vi "FilterSet.vi"(8 "error in (no error)":errorcluster caption="错误输入（无错误）", 11 "ParamIn":cluster{"mode":u8, "AccCode":u32, "AccMask":u32}={"mode"=1, "AccCode"=0, "AccMask"=4294967295} {"AccMask" format="%08x"; "AccCode" format="%08x"; "mode" items=["接收所有类型"=1, "只接收标准帧"=2, "只接收扩展帧"=3]}) -> (0 "error out":errorcluster caption="错误输出", 2 "Cancel？":bool, 3 "ParamOut":cluster{"mode":u8, "AccCode":u32, "AccMask":u32}={"mode"=1, "AccCode"=0, "AccMask"=0} {"AccMask" format="%08x"; "AccCode" format="%08x"; "mode" items=["接收所有类型"=1, "只接收标准帧"=2, "只接收扩展帧"=3]})   [LabVIEW 2011]
doc: "ID=0x6006"
panel:
  out "label2":string="CAN中继状态"
  in  "calc":bool
  in  "cancel":bool
  in  "ok":bool
  in  "AccMask":u32 caption="ÆÁ±Î´a£º0x" format="%08x"
  in  "AccCode":u32 caption="òžÊÕ´a£º0x" format="%08x"
  in  "mode":u8(ring)=1 caption="濾波方式:" items=["接收所有類型"=1, "Ö»ÊÕ˜ËœÊŽ¬"=2, "Ö»ÊÕ”UÕ¹Ž¬"=3]
  in  "selfdef":bool
  out "tab":enum32{"标准ID", "扩展ID", "全ID"}(tab)
  in  "ID00":bool
  in  "ID01":bool
  in  "ID02":bool
  in  "ID03":bool
  in  "ID04":bool
  in  "ID05":bool
  in  "ID06":bool
  in  "ID07":bool
  in  "ID08":bool
  in  "ID09":bool
  in  "ID10":bool
  in  "t1":i32(listbox)=-1
  in  "EID17":bool
  in  "EID16":bool
  in  "EID15":bool
  in  "EID14":bool
  in  "EID13":bool
  in  "EID12":bool
  in  "EID11":bool
  in  "EID10":bool
  in  "EID09":bool
  in  "EID08":bool
  in  "EID07":bool
  in  "EID06":bool
  in  "EID05":bool
  in  "EID04":bool
  in  "EID03":bool
  in  "EID02":bool
  in  "EID01":bool
  in  "EID00":bool
  in  "EID26":bool
  in  "EID25":bool
  in  "EID24":bool
  in  "EID23":bool
  in  "EID22":bool
  in  "EID21":bool
  in  "EID20":bool
  in  "EID19":bool
  in  "EID18":bool
  in  "EID27":bool
  in  "EID28":bool
  in  "t2":i32(listbox)=-1
  in  "ID10 2":bool
  in  "ID09 2":bool
  in  "ID08 2":bool
  in  "ID07 2":bool
  in  "ID06 2":bool
  in  "ID05 2":bool
  in  "ID04 2":bool
  in  "ID03 2":bool
  in  "ID02 2":bool
  in  "ID01 2":bool
  in  "ID00 2":bool
  in  "EID17 2":bool
  in  "EID16 2":bool
  in  "EID15 2":bool
  in  "EID14 2":bool
  in  "EID13 2":bool
  in  "EID12 2":bool
  in  "EID11 2":bool
  in  "EID10 2":bool
  in  "EID09 2":bool
  in  "EID08 2":bool
  in  "EID07 2":bool
  in  "EID06 2":bool
  in  "EID05 2":bool
  in  "EID04 2":bool
  in  "EID03 2":bool
  in  "EID02 2":bool
  in  "EID01 2":bool
  in  "EID00 2":bool
  in  "EID26 2":bool
  in  "EID25 2":bool
  in  "EID24 2":bool
  in  "EID23 2":bool
  in  "EID22 2":bool
  in  "EID21 2":bool
  in  "EID20 2":bool
  in  "EID19 2":bool
  in  "EID18 2":bool
  in  "EID27 2":bool
  in  "EID28 2":bool
  in  "t3":i32(listbox)=-1
  in  "Submit":bool
  in  "IDSet":u32 caption="指定ID：0x" format="%x"
  in  "FilterMode":u16(ring) caption="žV²¨Ä£Ê½ßx“ñ£º" items=["½ÓÊÕËùÓÐ”µ“þ", "˜ËœÊŽ¬žV²¨£¨ÔO¶¨½ÓÊÕ†Î‚€ID£©", "”UÕ¹Ž¬žV²¨£¨ÔO¶¨½ÓÊÕ†Î‚€ID£©", "˜ËœÊŽ¬žV²¨£¨ƒHID£¬×ÔÓÉÔO¶¨£©", "”UÕ¹Ž¬žV²¨£¨ƒHID£¬×ÔÓÉÔO¶¨£©"]
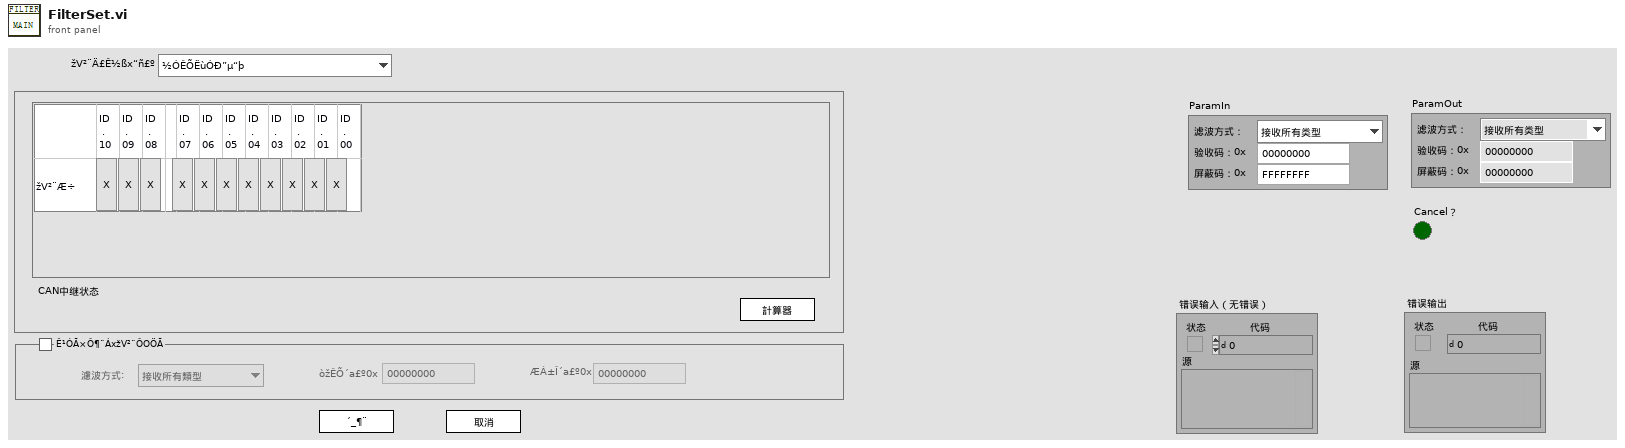
[diagram p1: front panel]
types:
  T1 = cluster{"FilterMode":refnum<vi>, "IDSet":refnum<vi>, "t1":refnum<vi>, "t2":refnum<vi>, "t3":refnum<vi>, "Submit":refnum<vi>, "tab":refnum<vi>, "calc":refnum<vi>, "selfdef":refnum<vi>, "mode":refnum<vi>, "AccCode":refnum<vi>, "AccMask":refnum<vi>, "ok":refnum<vi>, "cancel":refnum<vi>}
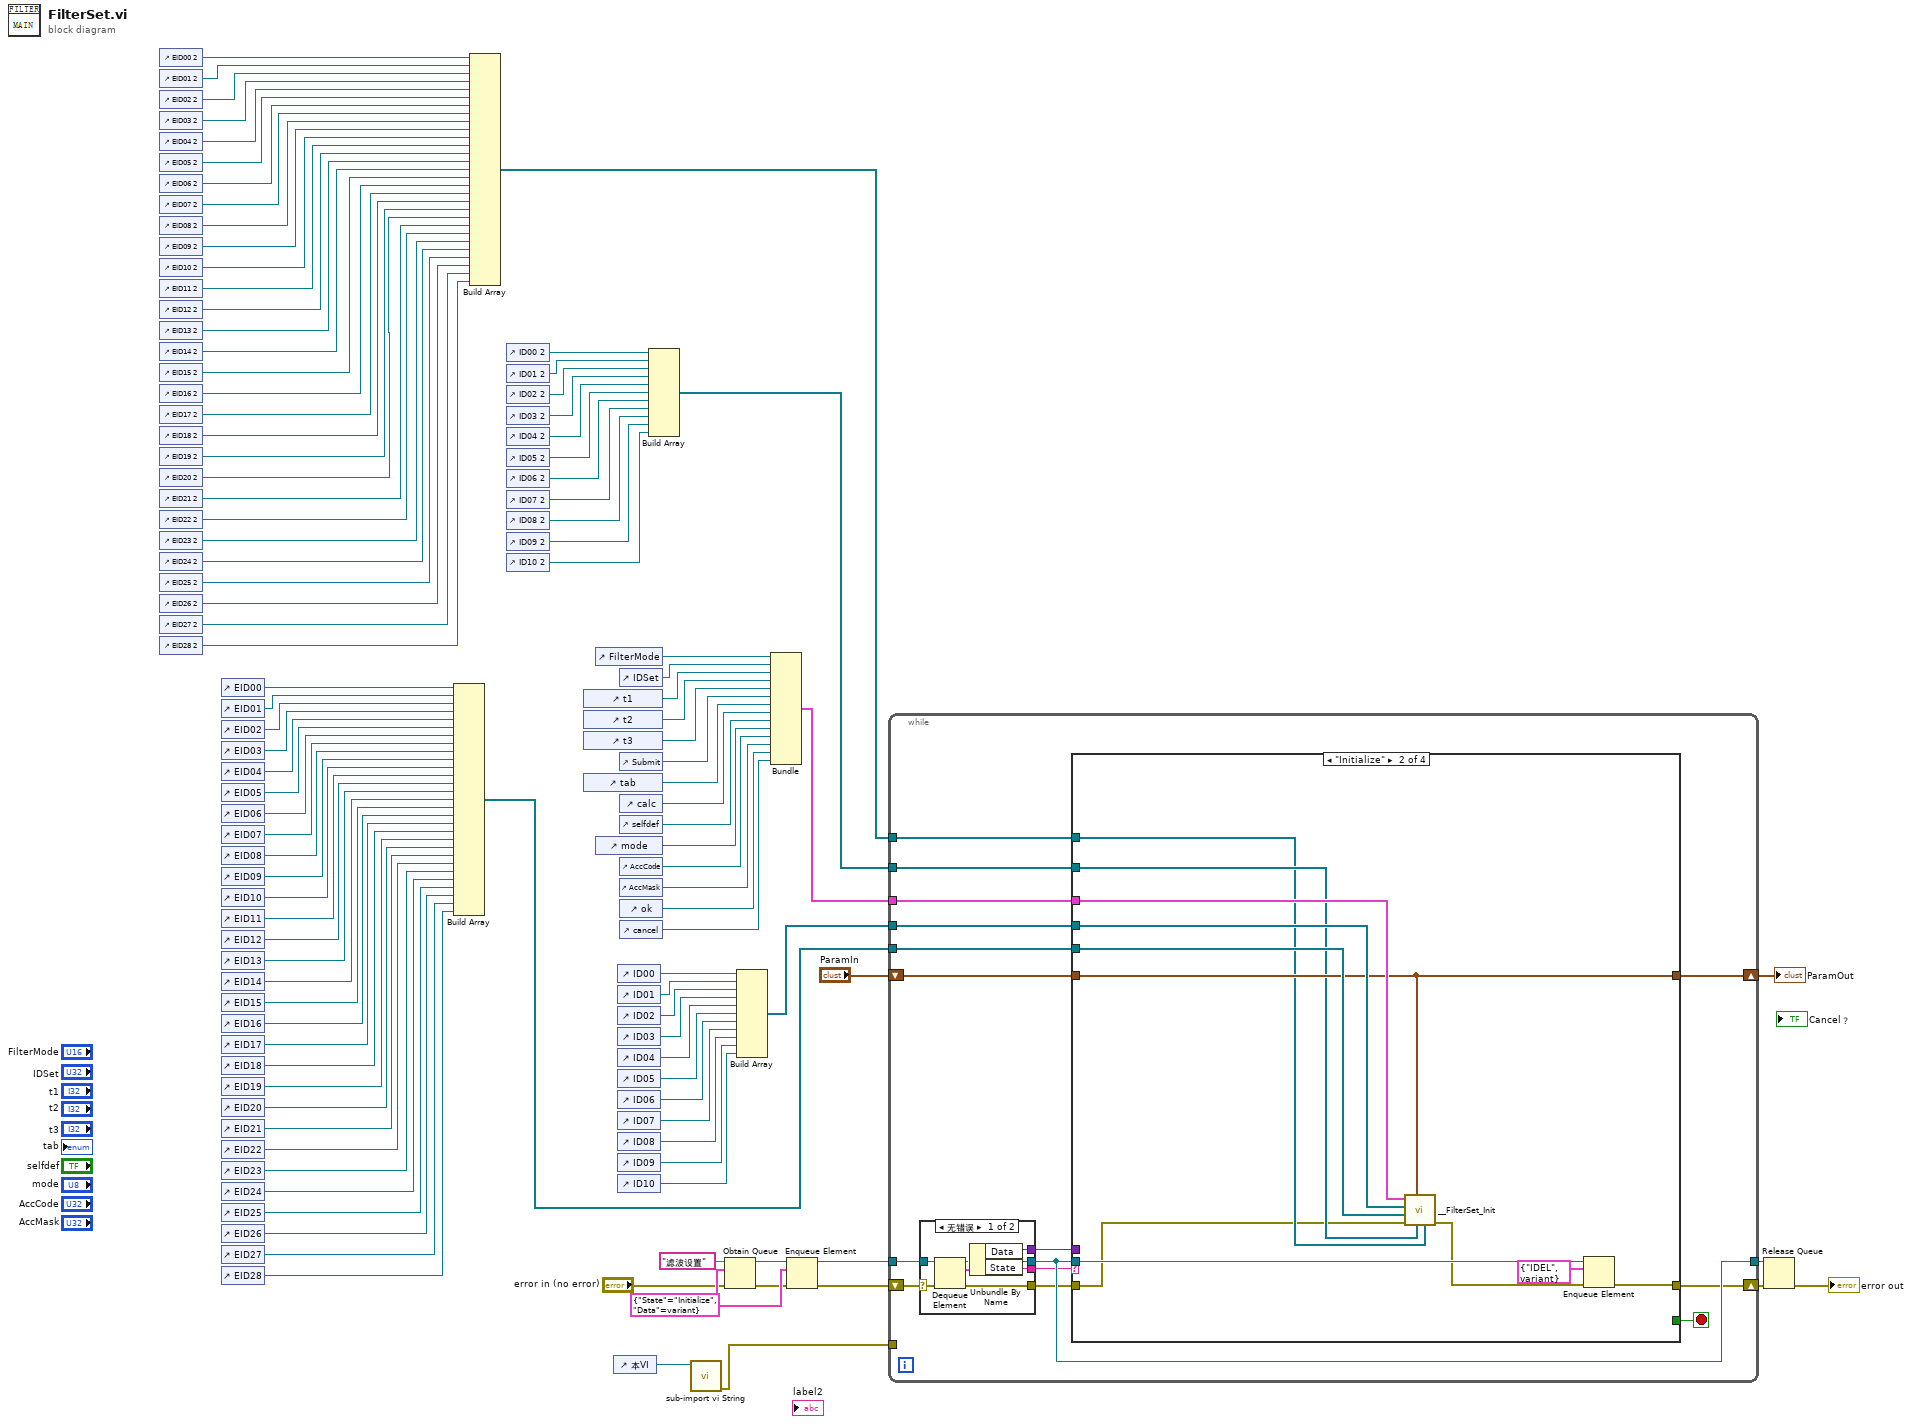
[diagram p0: block diagram]
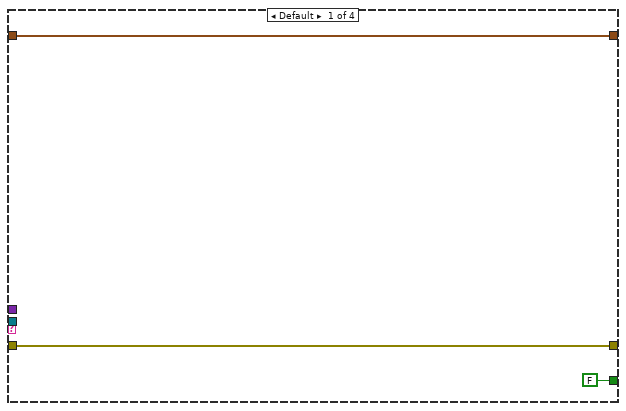
[diagram p2: hidden frame]
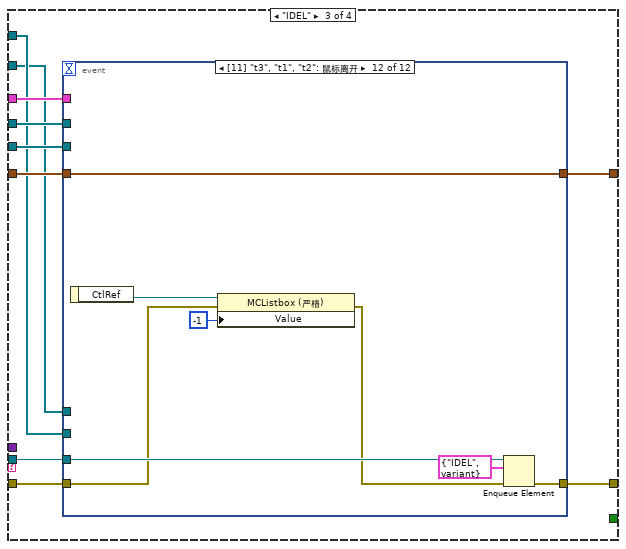
[diagram p3: hidden frame]
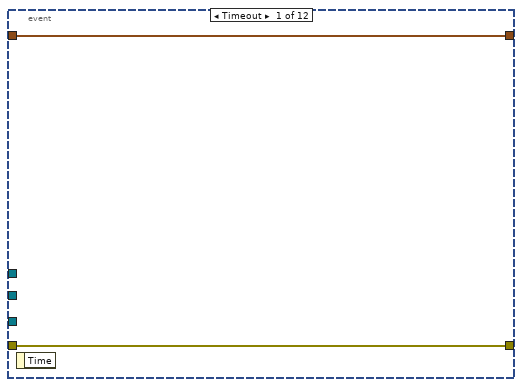
[diagram p4: hidden frame]
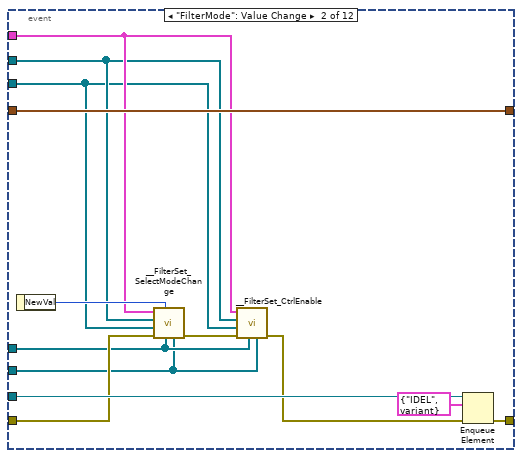
[diagram p5: hidden frame]
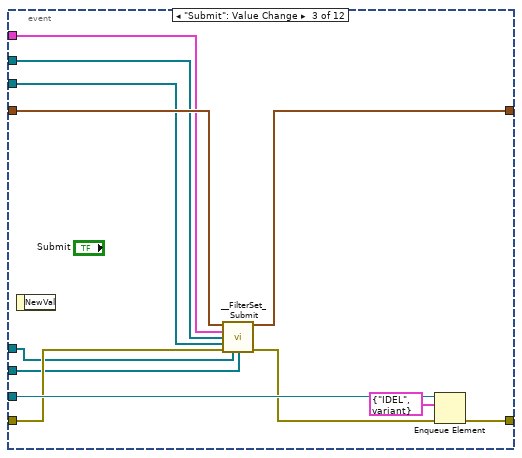
[diagram p6: hidden frame]
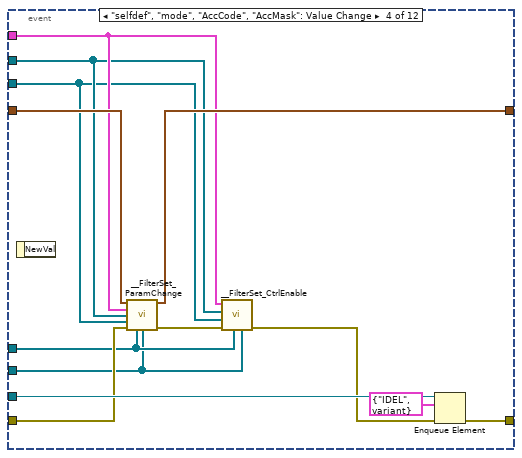
[diagram p7: hidden frame]
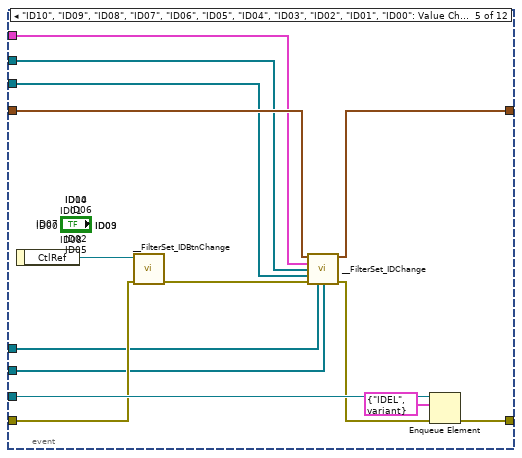
[diagram p8: hidden frame]
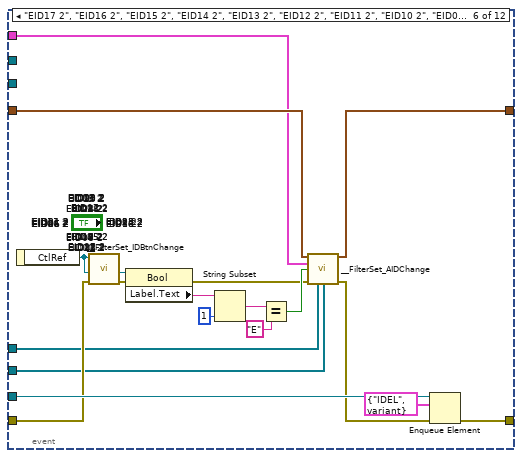
[diagram p9: hidden frame]
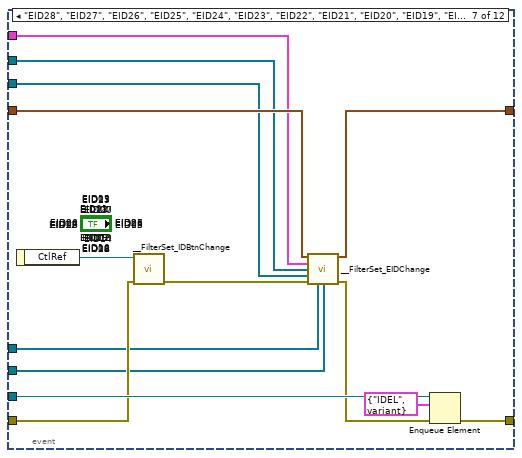
[diagram p10: hidden frame]
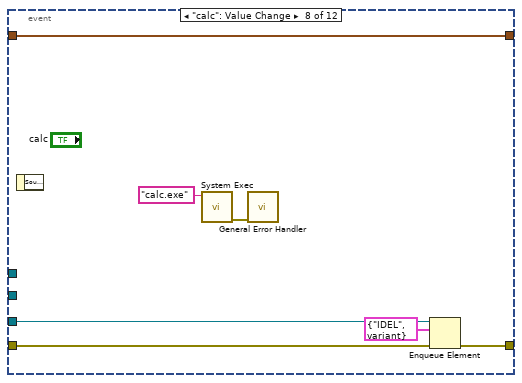
[diagram p11: hidden frame]
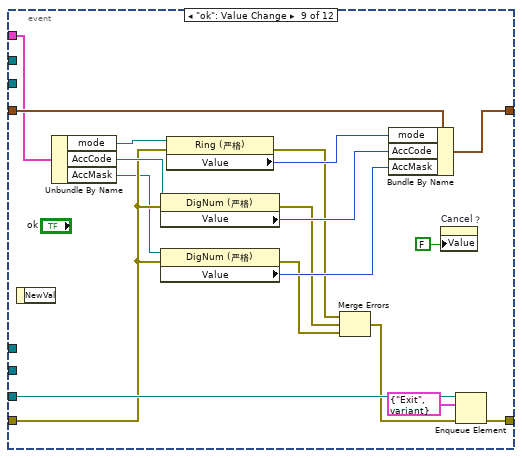
[diagram p12: hidden frame]
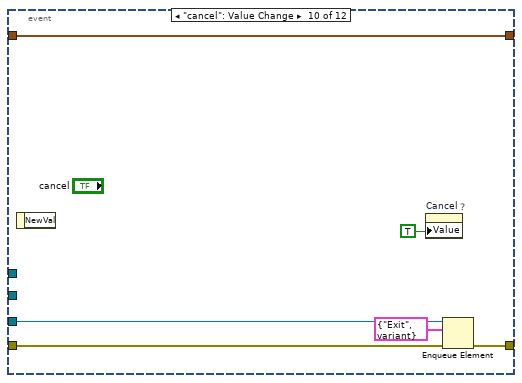
[diagram p13: hidden frame]
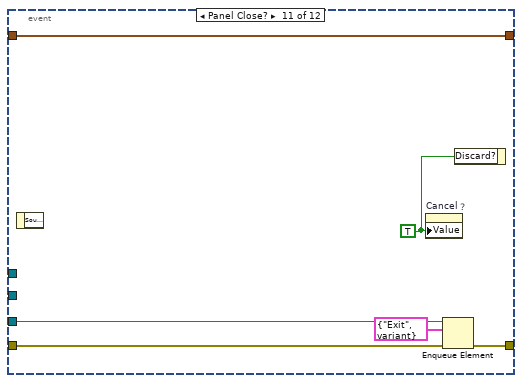
[diagram p14: hidden frame]
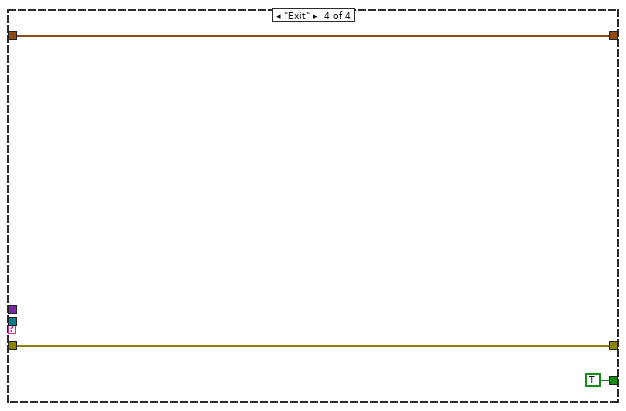
[diagram p15: hidden frame]
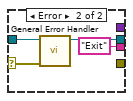
[diagram p16: hidden frame]
diagram:
  w113 = cluster{"State":string, "Data":variant} {"State"="Initialize", "Data"=variant}
  n1 = control-ref of="EID00 2"() -> (w47:refnum<vi>)
  n2 = control-ref of="EID01 2"() -> (w46:refnum<vi>)
  n3 = control-ref of="EID02 2"() -> (w45:refnum<vi>)
  n4 = control-ref of="EID03 2"() -> (w44:refnum<vi>)
  n5 = control-ref of="EID04 2"() -> (w43:refnum<vi>)
  n6 = control-ref of="EID05 2"() -> (w42:refnum<vi>)
  n7 = control-ref of="EID06 2"() -> (w41:refnum<vi>)
  n8 = control-ref of="EID07 2"() -> (w40:refnum<vi>)
  n9 = control-ref of="EID08 2"() -> (w39:refnum<vi>)
  n10 = control-ref of="EID09 2"() -> (w38:refnum<vi>)
  n11 = control-ref of="EID10 2"() -> (w37:refnum<vi>)
  n12 = control-ref of="EID11 2"() -> (w36:refnum<vi>)
  n13 = control-ref of="EID12 2"() -> (w35:refnum<vi>)
  n14 = control-ref of="EID13 2"() -> (w34:refnum<vi>)
  n15 = control-ref of="EID14 2"() -> (w33:refnum<vi>)
  n16 = control-ref of="EID15 2"() -> (w32:refnum<vi>)
  n17 = control-ref of="EID16 2"() -> (w31:refnum<vi>)
  n18 = control-ref of="EID17 2"() -> (w30:refnum<vi>)
  n19 = control-ref of="EID18 2"() -> (w29:refnum<vi>)
  n20 = control-ref of="EID19 2"() -> (w28:refnum<vi>)
  n21 = control-ref of="EID20 2"() -> (w27:refnum<vi>)
  n22 = control-ref of="EID21 2"() -> (w26:refnum<vi>)
  n23 = control-ref of="EID22 2"() -> (w25:refnum<vi>)
  n24 = control-ref of="EID23 2"() -> (w24:refnum<vi>)
  n25 = control-ref of="EID24 2"() -> (w23:refnum<vi>)
  n26 = control-ref of="EID25 2"() -> (w22:refnum<vi>)
  n27 = control-ref of="EID26 2"() -> (w21:refnum<vi>)
  n28 = control-ref of="EID27 2"() -> (w20:refnum<vi>)
  n29 = control-ref of="EID28 2"() -> (w19:refnum<vi>)
  n30 = control-ref of="EID00"() -> (w81:refnum<vi>)
  n31 = control-ref of="EID01"() -> (w80:refnum<vi>)
  n32 = control-ref of="EID02"() -> (w79:refnum<vi>)
  n33 = control-ref of="EID03"() -> (w78:refnum<vi>)
  n34 = control-ref of="EID04"() -> (w77:refnum<vi>)
  n35 = control-ref of="EID05"() -> (w76:refnum<vi>)
  n36 = control-ref of="EID06"() -> (w75:refnum<vi>)
  n37 = control-ref of="EID07"() -> (w74:refnum<vi>)
  n38 = control-ref of="EID08"() -> (w73:refnum<vi>)
  n39 = control-ref of="EID09"() -> (w72:refnum<vi>)
  n40 = control-ref of="EID10"() -> (w71:refnum<vi>)
  n41 = control-ref of="EID11"() -> (w70:refnum<vi>)
  n42 = control-ref of="EID12"() -> (w69:refnum<vi>)
  n43 = control-ref of="EID13"() -> (w68:refnum<vi>)
  n44 = control-ref of="EID14"() -> (w67:refnum<vi>)
  n45 = control-ref of="EID15"() -> (w66:refnum<vi>)
  n46 = control-ref of="EID16"() -> (w65:refnum<vi>)
  n47 = control-ref of="EID17"() -> (w64:refnum<vi>)
  n48 = control-ref of="EID18"() -> (w63:refnum<vi>)
  n49 = control-ref of="EID19"() -> (w62:refnum<vi>)
  n50 = control-ref of="EID20"() -> (w61:refnum<vi>)
  n51 = control-ref of="EID21"() -> (w60:refnum<vi>)
  n52 = control-ref of="EID22"() -> (w59:refnum<vi>)
  n53 = control-ref of="EID23"() -> (w58:refnum<vi>)
  n54 = control-ref of="EID24"() -> (w57:refnum<vi>)
  n55 = control-ref of="EID25"() -> (w56:refnum<vi>)
  n56 = control-ref of="EID26"() -> (w55:refnum<vi>)
  n57 = control-ref of="EID27"() -> (w54:refnum<vi>)
  n58 = control-ref of="EID28"() -> (w53:refnum<vi>)
  n59 = Build Array(w81, w80, w79, w78, w77, w76, w75, w74, w73, w72, w71, w70, w69, w68, w67, w66, w65, w64, w63, w62, w61, w60, w59, w58, w57, w56, w55, w54, w53) -> (w50:refnum<vi>[])
  n60 = Build Array(w47, w46, w45, w44, w43, w42, w41, w40, w39, w38, w37, w36, w35, w34, w33, w32, w31, w30, w29, w28, w27, w26, w25, w24, w23, w22, w21, w20, w19) -> (w7:refnum<vi>[])
  n61 = control-ref of="ID00 2"() -> (w18:refnum<vi>)
  n62 = control-ref of="ID01 2"() -> (w17:refnum<vi>)
  n63 = control-ref of="ID02 2"() -> (w16:refnum<vi>)
  n64 = control-ref of="ID03 2"() -> (w15:refnum<vi>)
  n65 = control-ref of="ID04 2"() -> (w14:refnum<vi>)
  n66 = control-ref of="ID05 2"() -> (w13:refnum<vi>)
  n67 = control-ref of="ID06 2"() -> (w12:refnum<vi>)
  n68 = control-ref of="ID07 2"() -> (w11:refnum<vi>)
  n69 = control-ref of="ID08 2"() -> (w10:refnum<vi>)
  n70 = control-ref of="ID09 2"() -> (w9:refnum<vi>)
  n71 = control-ref of="ID10 2"() -> (w8:refnum<vi>)
  n72 = control-ref of="t1"() -> (w103:refnum<vi>)
  n73 = control-ref of="t2"() -> (w102:refnum<vi>)
  n74 = control-ref of="t3"() -> (w5:refnum<vi>)
  n75 = control-ref of="tab"() -> (w100:refnum<vi>)
  n76 = control-ref of="FilterMode"() -> (w105:refnum<vi>)
  n77 = control-ref of="mode"() -> (w97:refnum<vi>)
  n78 = control-ref of="本VI"() -> (w1:refnum<vi>)
  n79 = control-ref of="ID00"() -> (w92:refnum<vi>)
  n80 = control-ref of="ID01"() -> (w91:refnum<vi>)
  n81 = control-ref of="ID02"() -> (w90:refnum<vi>)
  n82 = control-ref of="ID03"() -> (w89:refnum<vi>)
  n83 = control-ref of="ID04"() -> (w88:refnum<vi>)
  n84 = control-ref of="ID05"() -> (w87:refnum<vi>)
  n85 = control-ref of="ID06"() -> (w86:refnum<vi>)
  n86 = control-ref of="ID07"() -> (w85:refnum<vi>)
  n87 = control-ref of="ID08"() -> (w84:refnum<vi>)
  n88 = control-ref of="ID09"() -> (w83:refnum<vi>)
  n89 = control-ref of="ID10"() -> (w82:refnum<vi>)
  n90 = control-ref of="IDSet"() -> (w104:refnum<vi>)
  n91 = control-ref of="Submit"() -> (w101:refnum<vi>)
  n92 = control-ref of="calc"() -> (w99:refnum<vi>)
  n93 = control-ref of="selfdef"() -> (w98:refnum<vi>)
  n94 = control-ref of="AccCode"() -> (w96:refnum<vi>)
  n95 = control-ref of="AccMask"() -> (w95:refnum<vi>)
  n96 = control-ref of="ok"() -> (w94:refnum<vi>)
  n97 = control-ref of="cancel"() -> (w93:refnum<vi>)
  n98 = Build Array(w18, w17, w16, w15, w14, w13, w12, w11, w10, w9, w8) -> (w6:refnum<vi>[])
  n99 = call "sub-import vi String.vi"("vi ref"=w1) -> ("error out"=w2:errorcluster)  [unwired: 10 in]
  n100 = Obtain Queue(name (unnamed)="滤波设置", element data type=w113, error in (no error)="error in (no error)") -> (queue out=w111:refnum<queue>, error out=w112:errorcluster)  [unwired: 2 in, 1 out]
  n101 = Build Array(w92, w91, w90, w89, w88, w87, w86, w85, w84, w83, w82) -> (w51:refnum<vi>[])
  n102 = Bundle("FilterMode"=w105, "IDSet"=w104, "t1"=w103, "t2"=w102, "t3"=w5, "Submit"=w101, "tab"=w100, "calc"=w99, "selfdef"=w98, "mode"=w97, "AccCode"=w96, "AccMask"=w95, "ok"=w94, "cancel"=w93) -> (w52:T1)  [unwired: 1 in]
  n103 = Enqueue Element(queue=w111, element=w113, error in (no error)=w112) -> (queue out=w108:refnum<queue>, error out=w109:errorcluster)  [unwired: 2 out]
  n104 = while {
    shift-right: [w123] -> w107
    shift-left: w109 -> [w127]
    tunnel: w108 -> [w126]
    tunnel: [w128] -> w106
    tunnel: w52 -> [w121]
    tunnel: w51 -> [w120]
    tunnel: w50 -> [w119]
    shift-right: [w118] -> w49
    shift-left: "ParamIn" -> [w117]
    tunnel: w7 -> [w115]
    tunnel: w6 -> [w114]
    tunnel: w2 -> [_]
    stop <- w122 stop-if-true
    n105 = case shown="无错误" w127 {
      selector: w127 -> [w292 w296]
      tunnel: w126 -> [w293 w295]
      tunnel: [w288 "Exit" ("State")] -> w125
      tunnel: [w290 _] -> w124
      tunnel: [w289 w295] -> w128
      tunnel: [w287 _] -> w116
      frame No Error {
        n106 = Dequeue Element(queue=w293, error in (no error)=w292) -> (queue out=w289:refnum<queue>, element=w291:cluster{"State":string, "Data":variant}, error out=w290:errorcluster)  [unwired: 2 out]
        n107 = Unbundle By Name(w291) -> ("Data"=w287:variant, "State"=w288:string)
      }
      frame Error {
        n108 = call <vilib>:"General Error Handler.vi"("error in (no error)"=w296) -> ()  [unwired: 1 in, 14 out]
      }
    }
    n109 = case shown="\"Initialize\"" w125 {
      tunnel: w124 -> [w131 w132 w152 w286]
      tunnel: [w131 w140 w151 w286] -> w123
      tunnel: [FALSE _ _ TRUE] -> w122
      tunnel: w128 -> [_ w141 w150 _]
      tunnel: w121 -> [_ w139 w149 _]
      tunnel: w120 -> [_ w138 w148 _]
      tunnel: w119 -> [_ w137 w147 _]
      tunnel: [w129 w136 w145 w284] -> w118
      tunnel: w117 -> [w129 w136 w146 w284]
      tunnel: w116 -> [_ _ _ _]
      tunnel: w115 -> [_ w133 w144 _]
      tunnel: w114 -> [_ w134 w143 _]
      frame Default {
      }
      frame "Initialize" {
        n110 = call "__FilterSet_Init.vi"("EIDRef 2"=w133, "IDRef 2"=w134, "ParamIn"=w136, "error in (no error)"=w132, "EIDRef"=w137, "IDRef"=w138, "CtrlRef"=w139) -> ("error out"=w135:errorcluster)  [unwired: 4 in]
        n111 = Enqueue Element(queue=w141, element=cluster{"State":string, "Data":variant} {"State"="IDEL", "Data"=variant}, error in (no error)=w135) -> (error out=w140:errorcluster)  [unwired: 3 out]
      }
      frame "IDEL" {
        n112 = event shown="[11] \"t3\", \"t1\", \"t2\": 鼠标离开" {
          selector: _ -> [_ _ _ _ _ _ _ _ _ _ _ _]
          dyn-events: _ -> [_ _ _ _ _ _ _ _ _ _ _ _]
          timeout: _ -> [_ _ _ _ _ _ _ _ _ _ _ _]
          tunnel: w152 -> [w154 w164 w176 w187 w196 w217 w228 w240 w252 w266 w272 w278]
          tunnel: [w154 w166 w178 w191 w205 w223 w237 w244 w262 w267 w273 w281] -> w151
          tunnel: w150 -> [_ w167 w177 w190 w204 w222 w236 w243 w261 w265 w271 w280]
          tunnel: w149 -> [_ w159 w172 w184 w200 w218 w232 _ w257 _ _ _]
          tunnel: w148 -> [_ w158 w171 w183 w199 _ w231 _ _ _ _ _]
          tunnel: w147 -> [_ w157 w170 w182 w198 _ w230 _ _ _ _ _]
          tunnel: w146 -> [w153 w162 w174 w186 w203 w221 w235 w242 w259 w269 w275 w283]
          tunnel: [w153 w162 w173 w185 w202 w220 w234 w242 w258 w269 w275 w283] -> w145
          tunnel: w144 -> [_ w155 w168 w180 w193 w215 w225 _ _ _ _ _]
          tunnel: w143 -> [_ w156 w169 w181 w194 w216 w226 _ _ _ _ _]
          event Timeout {
            n113 = event-data() -> ()  [unwired: 1 in, 1 out]
          }
          event "FilterMode": Value Change {
            n114 = event-data() -> ("NewVal"=w163:u16)  [unwired: 1 in]
            n115 = call "__FilterSet_SelectModeChange.vi"("EIDRef 2"=w155, "IDRef 2"=w156, "Mode"=w163, "error in (no error)"=w164, "EIDRef"=w157, "IDRef"=w158, "CtrlRef"=w159) -> ("error out"=w161:errorcluster)  [unwired: 4 in]
            n116 = call "__FilterSet_CtrlEnable.vi"("EIDRef 2"=w155, "IDRef 2"=w156, "error in (no error)"=w161, "EIDRef"=w157, "IDRef"=w158, "CtrlRef"=w159) -> ("error out"=w160:errorcluster)  [unwired: 5 in]
            n117 = Enqueue Element(queue=w167, element=cluster{"State":string, "Data":variant} {"State"="IDEL", "Data"=variant}, error in (no error)=w160) -> (error out=w166:errorcluster)  [unwired: 3 out]
          }
          event "Submit": Value Change {
            n118 = event-data() -> ()  [unwired: 1 in, 1 out]
            n119 = call "__FilterSet_Submit.vi"("Param in"=w174, "CtrlRef"=w172, "IDRef"=w171, "EIDRef"=w170, "error in (no error)"=w176, "IDRef 2"=w169, "EIDRef 2"=w168) -> ("Param out"=w173:cluster{"mode":u8, "AccCode":u32, "AccMask":u32}, "error out"=w175:errorcluster)  [unwired: 7 in]
            n120 = Enqueue Element(queue=w177, element=cluster{"State":string, "Data":variant} {"State"="IDEL", "Data"=variant}, error in (no error)=w175) -> (error out=w178:errorcluster)  [unwired: 3 out]
          }
          event "selfdef", "mode", "AccCode", "AccMask": Value Change {
            n121 = event-data() -> ()  [unwired: 1 in, 1 out]
            n122 = call "__FilterSet_ParamChange.vi"("Param in"=w186, "CtrlRef"=w184, "IDRef"=w183, "EIDRef"=w182, "error in (no error)"=w187, "IDRef 2"=w181, "EIDRef 2"=w180) -> ("Param out"=w185:cluster{"mode":u8, "AccCode":u32, "AccMask":u32}, "error out"=w188:errorcluster)  [unwired: 7 in]
            n123 = call "__FilterSet_CtrlEnable.vi"("EIDRef 2"=w180, "IDRef 2"=w181, "error in (no error)"=w188, "EIDRef"=w182, "IDRef"=w183, "CtrlRef"=w184) -> ("error out"=w189:errorcluster)  [unwired: 5 in]
            n124 = Enqueue Element(queue=w190, element=cluster{"State":string, "Data":variant} {"State"="IDEL", "Data"=variant}, error in (no error)=w189) -> (error out=w191:errorcluster)  [unwired: 3 out]
          }
          event "ID10", "ID09", "ID08", "ID07", "ID06", "ID05", "ID04", "ID03", "ID02", "ID01", "ID00": Value Change {
            n125 = event-data() -> ("CtlRef"=w197:refnum<vi>)  [unwired: 1 in]
            n126 = call "__FilterSet_IDBtnChange.vi"("error in (no error)"=w196, "Btn Ref"=w197) -> ("error out"=w195:errorcluster)  [unwired: 9 in]
            n127 = call "__FilterSet_IDChange.vi"("Param in"=w203, "CtrlRef"=w200, "IDRef"=w199, "EIDRef"=w198, "error in (no error)"=w195, "IDRef 2"=w194, "EIDRef 2"=w193) -> ("Param out"=w202:cluster{"mode":u8, "AccCode":u32, "AccMask":u32}, "error out"=w201:errorcluster)  [unwired: 7 in]
            n128 = Enqueue Element(queue=w204, element=cluster{"State":string, "Data":variant} {"State"="IDEL", "Data"=variant}, error in (no error)=w201) -> (error out=w205:errorcluster)  [unwired: 3 out]
          }
          event "EID17 2", "EID16 2", "EID15 2", "EID14 2", "EID13 2", "EID12 2", "EID11 2", "EID10 2", "EID09 2", "EID08 2", "EID07 2", "EID06 2", "EID05 2", "EID04 2", "EID03 2", "EID02 2", "EID01 2", "EID00 2", "EID26 2", "EID25 2", "EID24 2", "EID23 2", "EID22 2", "EID21 2", "EID20 2", "EID19 2", "EID18 2", "EID27 2", "EID28 2", "ID10 2", "ID09 2", "ID08 2", "ID07 2", "ID06 2", "ID05 2", "ID04 2", "ID03 2", "ID02 2", "ID01 2", "ID00 2": Value Change {
            n129 = event-data() -> ("CtlRef"=w207:refnum<vi>)  [unwired: 1 in]
            n130 = call "__FilterSet_IDBtnChange.vi"("error in (no error)"=w217, "Btn Ref"=w207) -> ("error out"=w214:errorcluster)  [unwired: 9 in]
            n131 = property class="Bool"(reference=w207, error in=w214) -> (error out=w208:errorcluster, "Label.Text"=w213:string)  [unwired: 1 out]
            n132 = String Subset(string=w213, length (rest)=1 ("长度（剩余）")) -> (substring=w211:string)  [unwired: 1 in]
            n133 = Equal?(x=w211, y="E") -> (x = y?=w209:bool)
            n134 = call "__FilterSet_AIDChange.vi"("Param in"=w221, "CtrlRef"=w218, "EID?"=w209, "error in (no error)"=w208, "IDRef 2"=w216, "EIDRef 2"=w215) -> ("Param out"=w220:cluster{"mode":u8, "AccCode":u32, "AccMask":u32}, "error out"=w219:errorcluster)  [unwired: 8 in]
            n135 = Enqueue Element(queue=w222, element=cluster{"State":string, "Data":variant} {"State"="IDEL", "Data"=variant}, error in (no error)=w219) -> (error out=w223:errorcluster)  [unwired: 3 out]
          }
          event "EID28", "EID27", "EID26", "EID25", "EID24", "EID23", "EID22", "EID21", "EID20", "EID19", "EID18", "EID17", "EID16", "EID15", "EID14", "EID13", "EID12", "EID11", "EID10", "EID09", "EID08", "EID07", "EID06", "EID05", "EID04", "EID03", "EID02", "EID01", "EID00": Value Change {
            n136 = event-data() -> ("CtlRef"=w229:refnum<vi>)  [unwired: 1 in]
            n137 = call "__FilterSet_IDBtnChange.vi"("error in (no error)"=w228, "Btn Ref"=w229) -> ("error out"=w227:errorcluster)  [unwired: 9 in]
            n138 = call "__FilterSet_EIDChange.vi"("Param in"=w235, "CtrlRef"=w232, "IDRef"=w231, "EIDRef"=w230, "error in (no error)"=w227, "IDRef 2"=w226, "EIDRef 2"=w225) -> ("Param out"=w234:cluster{"mode":u8, "AccCode":u32, "AccMask":u32}, "error out"=w233:errorcluster)  [unwired: 7 in]
            n139 = Enqueue Element(queue=w236, element=cluster{"State":string, "Data":variant} {"State"="IDEL", "Data"=variant}, error in (no error)=w233) -> (error out=w237:errorcluster)  [unwired: 3 out]
          }
          event "calc": Value Change {
            n140 = event-data() -> ()  [unwired: 1 in, 1 out]
            n141 = call <vilib>:"System Exec.vi"("command line"="calc.exe") -> ("error out"=w239:errorcluster)  [unwired: 7 in, 3 out]
            n142 = call <vilib>:"General Error Handler.vi"("error in (no error)"=w239) -> ()  [unwired: 1 in, 14 out]
            n143 = Enqueue Element(queue=w243, element=cluster{"State":string, "Data":variant} {"State"="IDEL", "Data"=variant}, error in (no error)=w240) -> (error out=w244:errorcluster)  [unwired: 3 out]
          }
          event "ok": Value Change {
            n144 = event-data() -> ()  [unwired: 1 in, 1 out]
            n145 = Unbundle By Name(w257) -> ("mode"=w256:refnum<vi>, "AccCode"=w254:refnum<vi>, "AccMask"=w251:refnum<vi>)
            n146 = property class="DigNum (严格)"(reference=w254, error in=w252) -> (error out=w248:errorcluster, "Value"=w253:u32)  [unwired: 1 out]
            n147 = property class="DigNum (严格)"(reference=w251, error in=w252) -> (error out=w247:errorcluster, "Value"=w250:u32)  [unwired: 1 out]
            n148 = property class="Ring (严格)"(reference=w256, error in=w252) -> (error out=w249:errorcluster, "Value"=w255:u8)  [unwired: 1 out]
            n149 = Merge Errors(w249, w248, w247) -> (w246:errorcluster)
            n150 = Bundle By Name(cluster=w259, "mode"=w255, "AccCode"=w253, "AccMask"=w250) -> (w258:cluster{"mode":u8, "AccCode":u32, "AccMask":u32})
            n151 = property on="Cancel？" class="Bool (严格)"("Value"=FALSE ("Cancel？")) -> ()  [unwired: 2 in, 2 out]
            n152 = Enqueue Element(queue=w261, element=cluster{"State":string, "Data":variant} {"State"="Exit", "Data"=variant}, error in (no error)=w246) -> (error out=w262:errorcluster)  [unwired: 3 out]
          }
          event "cancel": Value Change {
            n153 = event-data() -> ()  [unwired: 1 in, 1 out]
            n154 = property on="Cancel？" class="Bool (严格)"("Value"=TRUE ("Cancel？")) -> ()  [unwired: 2 in, 2 out]
            n155 = Enqueue Element(queue=w265, element=cluster{"State":string, "Data":variant} {"State"="Exit", "Data"=variant}, error in (no error)=w266) -> (error out=w267:errorcluster)  [unwired: 3 out]
          }
          event Panel Close? {
            w270 = TRUE ("Cancel？")
            n156 = event-data() -> ()  [unwired: 1 in, 1 out]
            n157 = property on="Cancel？" class="Bool (严格)"("Value"=w270) -> ()  [unwired: 2 in, 2 out]
            n158 = Enqueue Element(queue=w271, element=cluster{"State":string, "Data":variant} {"State"="Exit", "Data"=variant}, error in (no error)=w272) -> (error out=w273:errorcluster)  [unwired: 3 out]
            n159 = event-data("Discard?"=w270) -> ()  [unwired: 1 in, 1 out]
          }
          event "t3", "t1", "t2": Mouse Leave {
            n160 = event-data() -> ("CtlRef"=w279:refnum<vi>)  [unwired: 1 in]
            n161 = property class="MCListbox (严格)"(reference=w279, error in=w278, "Value"=-1 ("值")) -> (error out=w277:errorcluster)  [unwired: 1 out]
            n162 = Enqueue Element(queue=w280, element=cluster{"State":string, "Data":variant} {"State"="IDEL", "Data"=variant}, error in (no error)=w277) -> (error out=w281:errorcluster)  [unwired: 3 out]
          }
        }
      }
      frame "Exit" {
      }
    }
  }
  "ParamOut" <- w49
  n163 = Release Queue(queue=w106, error in (no error)=w107) -> (error out=→"error out":errorcluster)  [unwired: 3 out]
